vi "Write configuration.vi"(8 "error in (no error)":errorcluster, 10 "configuration":refnum<class "CEF_serializable configuration.lvclass">, 11 "Abstract Digitizer":refnum<class "ACIR Instrument.lvclass">) -> (0 "error out":errorcluster, 3 "Abstract Digitizer out":refnum<class "ACIR Instrument.lvclass">)   [LabVIEW 2025, in "ACIR.lvlib" / "ACIR Instrument.lvclass"]
uses:
  ACIR Instrument.lvclass
  Users/Public/Documents/Sandia National Labs/TSS Plugin/CEF.lvlibp/serializable configuration/CEF_serializable configuration.lvclass
  ACIR configuration/ACIR configuration.lvclass
  ACIR Instrument.lvclass/ACIR Instrument.ctl
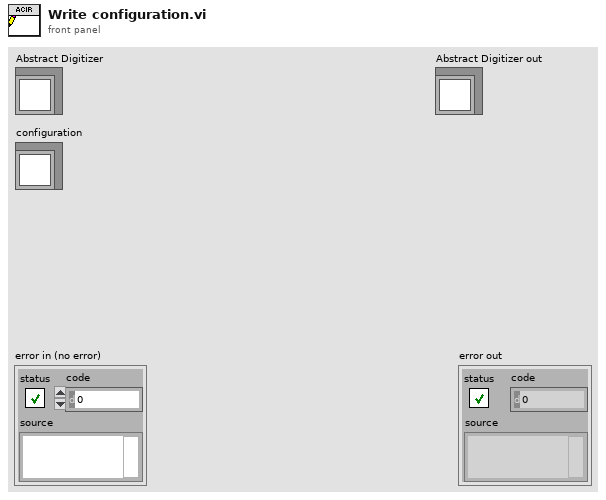
[diagram p1: front panel]
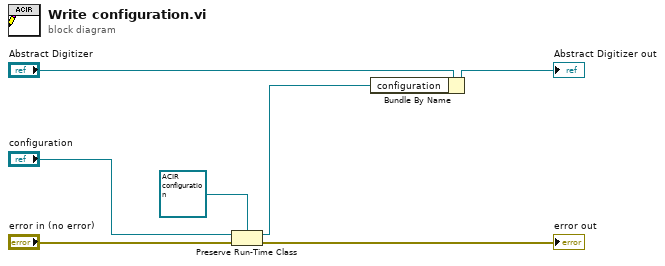
[diagram p0: block diagram]
diagram:
  n1 = Preserve Run-Time Class(object in="configuration", error in="error in (no error)", 2:refnum<class "ACIR configuration.lvclass"> refnum ("Digitizer.lvlib:Digitizer configuration.lvclass")) -> (object out=w4:refnum<class "ACIR configuration.lvclass">, error out=→"error out":errorcluster)
  n2 = Bundle By Name(cluster="Abstract Digitizer", "configuration"=w4) -> (→"Abstract Digitizer out":refnum<class "ACIR Instrument.lvclass">)
